vi "DangerEnemy.vi"(0 "MarkerSkill in":refnum<class "MarkerSkill.lvclass">, 5 "Game":refnum<class "Game.lvclass">, 11 "error in (no error)":errorcluster) -> (3 "Numero de inimigos\npossiveis para marcar":i32, 4 "MarkerSkill out":refnum<class "MarkerSkill.lvclass">, 6 "id do inimigo\nmais perigoso":u32, 8 "Pos do inimigo\nperigoso":dbl[](array[numeric]), 10 "id do segundo inimigo\nmais perigoso":i32, 13 "Id do Inimigo Mais Próximo":u32, 14 "Pos do segundo inimigo\nperigoso":dbl[](array[numeric]), 15 "error out":errorcluster)   [LabVIEW 2018, in "MarkerSkill.lvclass"]
uses:
  MarkerSkill.lvclass
  Game_class/Game.lvclass
  Game_class/Game.lvclass/Game.ctl
  Referee_class/Referee.lvclass/Referee.ctl
  Team_class/Team.lvclass/Team.ctl
  Object_class/Object.lvclass/Object.ctl
  Robot_class/Robot.lvclass/Robot.ctl
  Object_class/Read x.vi
  Object_class/Read y.vi
  Robot_class/Read id.vi
  <vilib>/Analysis/_algsub.llb/Real Vector Norm.vi
  Game_class/Read Referee.vi
  Game_class/Read EnemyRef.vi
  Game_class/Read FieldRef.vi
  Game_class/Read BallRef.vi
  Team_class/Read RobotRef.vi
  Referee_class/Read enemy_goalie_id.vi
  Enemy_class/Enemy.lvclass
  C:/Users/Gustavo/Desktop/RoboIME/SimplePass/SSL_AI/Team_class/Team.lvclass
  Ball_class/Ball.lvclass
  C:/Users/Gustavo/Desktop/RoboIME/SimplePass/SSL_AI/Object_class/Object.lvclass
  Robot_class/Robot.lvclass
  Referee_class/Referee.lvclass
  Field_class/Field.lvclass
  <vilib>/Analysis/NI_AALPro.lvlib
panel:
  in  "D para nao marcar":dbl=200.0
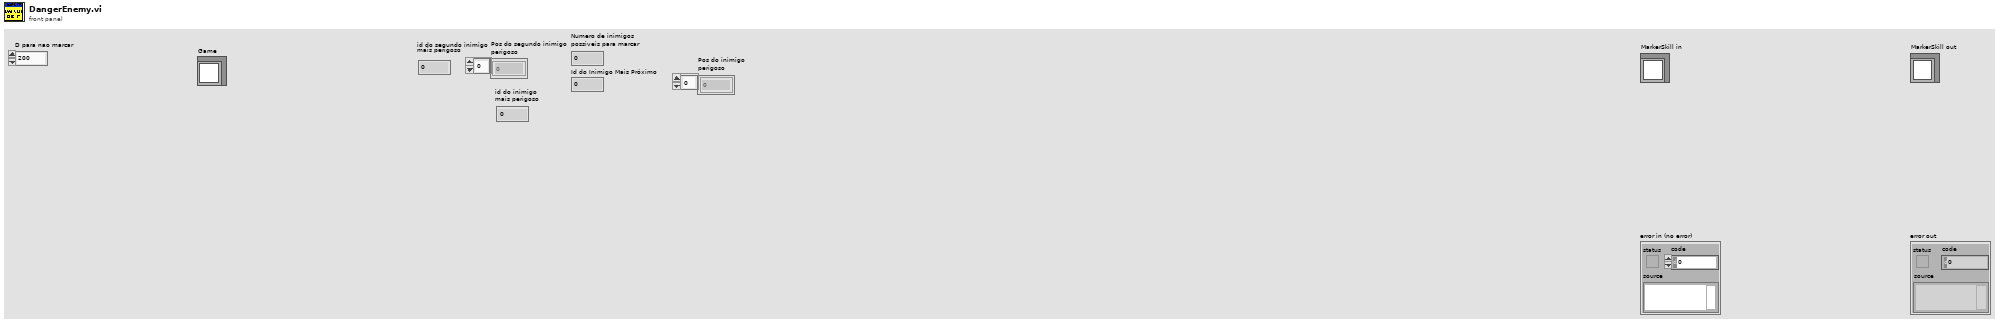
[diagram p1: front panel]
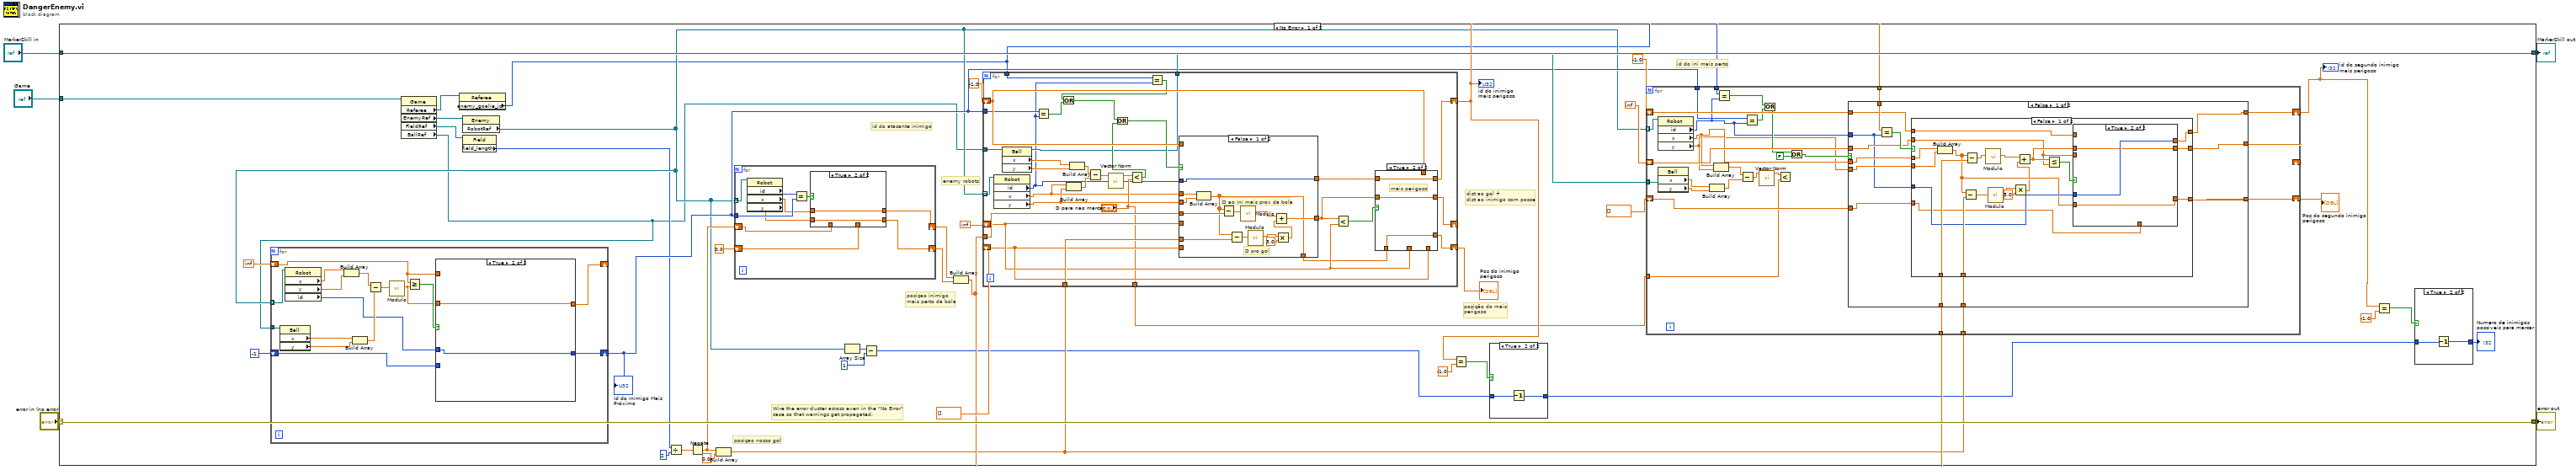
[diagram p0: block diagram]
diagram:
  n1 = case shown="No Error" "error in (no error)" {
    selector: "error in (no error)" -> [w47 w217]
    tunnel: [w47 w217] -> w4
    tunnel: [w48 w216] -> w2
    tunnel: "MarkerSkill in" -> [w48 w216]
    tunnel: "Game" -> [w6 _]
    frame No Error {
      # "id do ini mais perto"
      # "id do atacante inimigo"
      # "enemy robots"
      # "dist ao gol +\ndist ao inimigo com posse"
      # "posição do mais\nperigoso"
      # "posiçao nosso gol"
      # "posiçao inimigo\nmais perto da bola"
      # "Wire the error cluster across even in the \"No Error\"\ncase so that warnings get propagated."
      n2 = property class="Game"(reference=w6) -> ("Referee"=w8:refnum<class "Referee.lvclass">, "EnemyRef"=w13:refnum<class "Enemy.lvclass">, "FieldRef"=w12:refnum<class "Field.lvclass">, "BallRef"=w9:refnum<class "Ball.lvclass">)  [unwired: 1 in, 2 out]
      n3 = property class="Referee"(reference=w8) -> ("enemy_goalie_id"=w7:i32)  [unwired: 1 in, 2 out]
      n4 = property class="Enemy"(reference=w13) -> ("RobotRef"=w11:refnum<class "Robot.lvclass">[])  [unwired: 1 in, 2 out]
      n5 = for {
        tunnel: w11 -> [w58] mode=indexing
        tunnel: w9 -> [w61]
        shift-right: [w65] -> _
        shift-left: inf -> [w63]
        shift-right: [w64] -> w15
        shift-left: -1 -> [w62]
        n6 = property class="Ball"(reference=w61) -> ("x"=w60:dbl, "y"=w59:dbl)  [unwired: 1 in, 2 out]
        n7 = property class="Robot"(reference=w58) -> ("x"=w57:dbl, "y"=w56:dbl, "id"=w55:i32)  [unwired: 1 in, 2 out]
        n8 = Build Array(w57, w56) -> (w70:dbl[])
        n9 = Build Array(w60, w59) -> (w69:dbl[])
        n10 = Subtract(x=w70, y=w69) -> (x-y=w67:dbl[])
        n11 = call "Modulo.vi"("2D vector"=w67) -> ("Modulo"=w66:dbl)  [unwired: 10 in]
        n12 = Greater Or Equal?(x=w63, y=w66) -> (x >= y?=w68:bool)
        n13 = case shown="True" w68 {
          tunnel: [w72 w74] -> w65
          tunnel: w66 -> [_ w74]
          tunnel: w55 -> [_ w73]
          tunnel: [w71 w73] -> w64
          tunnel: w63 -> [w72 _]
          tunnel: w62 -> [w71 _]
          frame False {
          }
          frame True {
          }
        }
      }
      "Id do Inimigo Mais Próximo" <- w15
      n14 = property class="Field"(reference=w12) -> ("field_length"=w10:i32)  [unwired: 1 in, 2 out]
      n15 = Divide(x=w10, y=u32 2) -> (x/y=w44:dbl)
      n16 = Negate(x=w44) -> (-x=w39:dbl)
      n17 = Build Array(w39, 0.0 ("element")) -> (w33:dbl[])
      n18 = for {
        tunnel: w11 -> [w205] mode=indexing
        tunnel: w15 -> [w211]
        shift-right: [w209] -> w17
        shift-left: w39 -> [w207]
        shift-right: [w208] -> w46
        shift-left: 0.0 ("y") -> [w206]
        n19 = property class="Robot"(reference=w205) -> ("id"=w204:i32, "x"=w203:dbl, "y"=w202:dbl)  [unwired: 1 in, 2 out]
        n20 = Equal?(x=w204, y=w211) -> (x = y?=w210:bool)
        n21 = case shown="True" w210 {
          tunnel: w203 -> [_ w215]
          tunnel: w202 -> [_ w214]
          tunnel: [w213 w215] -> w209
          tunnel: [w212 w214] -> w208
          tunnel: w207 -> [w213 _]
          tunnel: w206 -> [w212 _]
          frame False {
          }
          frame True {
          }
        }
      }
      n22 = Array Size(array=w11) -> (size(s)=w30:i32)
      n23 = Subtract(x=w30, y=1) -> (x-y=w25:i32)
      n24 = Build Array(w17, w46) -> (w34:dbl[])
      n25 = for {
        tunnel: w11 -> [w151] mode=indexing
        tunnel: w34 -> [w179]
        tunnel: w33 -> [w178]
        shift-right: [w175] -> _
        shift-left: inf -> [w174]
        shift-right: [w172] -> w28
        shift-left: -1.0 ("id") -> [w169]
        shift-right: [w170] -> w42
        shift-left: dbl[] [] -> [w168]
        tunnel: w7 -> [w167]
        tunnel: w9 -> [w155]
        tunnel: [w152] -> w19
        tunnel: ["D para nao marcar"] -> w18
        tunnel: w15 -> [w157]
        n26 = property class="Robot"(reference=w151) -> ("id"=w148:i32, "x"=w150:dbl, "y"=w149:dbl)  [unwired: 1 in, 2 out]
        n27 = property class="Ball"(reference=w155) -> (reference out=w152:refnum<class "Ball.lvclass">, "x"=w154:dbl, "y"=w153:dbl)  [unwired: 1 in, 1 out]
        n28 = Equal?(x=w157, y=w148) -> (x = y?=w165:bool)
        n29 = Build Array(w150, w149) -> (w163:dbl[])
        n30 = Build Array(w154, w153) -> (w164:dbl[])
        n31 = Subtract(x=w164, y=w163) -> (x-y=w162:dbl[])
        n32 = call-poly <vilib>:"Vector Norm.vi"("Input Vector"=w162) -> ("norm"=w161:dbl)  [unwired: 9 in, 1 out]
        n33 = Less?(x=w161, y="D para nao marcar") -> (x < y?=w156:bool)
        n34 = Equal?(x=w167, y=w148) -> (x = y?=w166:bool)
        n35 = Or(x=w166, y=w165) -> (x .or. y?=w160:bool)
        n36 = Or(x=w160, y=w156) -> (x .or. y?=w159:bool)
        n37 = case shown="False" w159 {
          tunnel: w150 -> [w198 _]
          tunnel: w149 -> [w197 _]
          tunnel: w179 -> [w196 _]
          tunnel: w178 -> [w194 _]
          tunnel: [w191 w201] -> w176
          tunnel: w174 -> [_ w201]
          tunnel: w148 -> [w190 _]
          tunnel: [w190 w200] -> w173
          tunnel: [w189 w199] -> w171
          tunnel: w169 -> [_ w200]
          tunnel: w168 -> [_ w199]
          frame False {
            # "D ao ini mais prox da bola"
            # "D pro gol"
            n38 = Build Array(w198, w197) -> (w189:dbl[])
            n39 = Subtract(x=w189, y=w196) -> (x-y=w195:dbl[])
            n40 = Subtract(x=w189, y=w194) -> (x-y=w193:dbl[])
            n41 = call "Modulo.vi"("2D vector"=w195) -> ("Modulo"=w192:dbl)  [unwired: 10 in]
            n42 = call "Modulo.vi"("2D vector"=w193) -> ("Modulo"=w188:dbl)  [unwired: 10 in]
            n43 = Multiply(x=w188, y=3.0) -> (x*y=w186:dbl)
            n44 = Add(x=w192, y=w186) -> (x+y=w191:dbl)
          }
          frame True {
          }
        }
        n45 = Less?(x=w176, y=w174) -> (x < y?=w177:bool)
        n46 = case shown="True" w177 {
          tunnel: w176 -> [_ w185]
          tunnel: [w182 w185] -> w175
          tunnel: w174 -> [w182 _]
          tunnel: [w181 w184] -> w172
          tunnel: w173 -> [_ w184]
          tunnel: w169 -> [w181 _]
          tunnel: w171 -> [_ w183]
          tunnel: [w180 w183] -> w170
          tunnel: w168 -> [w180 _]
          frame False {
          }
          frame True {
            # "mais perigoso"
          }
        }
      }
      "id do inimigo\nmais perigoso" <- w28
      "Pos do inimigo\nperigoso" <- w42
      n47 = Equal?(x=w28, y=-1.0) -> (x = y?=w26:bool)
      n48 = case shown="True" w26 {
        tunnel: w25 -> [w52 w54]
        tunnel: [w52 w53] -> w21
        frame False {
        }
        frame True {
          n49 = Decrement(x=w54) -> (x-1=w53:i32)
        }
      }
      n50 = for {
        tunnel: w11 -> [w81] mode=indexing
        shift-right: [w102] -> w23
        shift-left: -1.0 -> [w101]
        shift-right: [w100] -> _
        shift-left: inf -> [w94]
        shift-right: [w99] -> w35
        shift-left: dbl[] [] -> [w98]
        tunnel: w28 -> [w97]
        tunnel: w34 -> [w96]
        tunnel: w33 -> [w95]
        tunnel: w7 -> [w93]
        tunnel: w19 -> [w77]
        tunnel: w18 -> [w86]
        tunnel: w15 -> [w83]
        n51 = property class="Robot"(reference=w81) -> ("id"=w80:i32, "x"=w79:dbl, "y"=w78:dbl)  [unwired: 1 in, 2 out]
        n52 = property class="Ball"(reference=w77) -> ("x"=w76:dbl, "y"=w75:dbl)  [unwired: 1 in, 2 out]
        n53 = Build Array(w76, w75) -> (w89:dbl[])
        n54 = Build Array(w79, w78) -> (w90:dbl[])
        n55 = Equal?(x=w93, y=w80) -> (x = y?=w92:bool)
        n56 = Subtract(x=w90, y=w89) -> (x-y=w88:dbl[])
        n57 = Equal?(x=w83, y=w80) -> (x = y?=w91:bool)
        n58 = call-poly <vilib>:"Vector Norm.vi"("Input Vector"=w88) -> ("norm"=w87:dbl)  [unwired: 9 in, 1 out]
        n59 = Or(x=w92, y=w91) -> (x .or. y?=w85:bool)
        n60 = Less?(x=w87, y=w86) -> ()  [unwired: 1 out]
        n61 = Or(x=w85, y=FALSE) -> (x .or. y?=w84:bool)
        n62 = case shown="False" w84 {
          tunnel: w101 -> [w113 w147]
          tunnel: [w112 w147] -> w102
          tunnel: w94 -> [w111 w146]
          tunnel: [w110 w146] -> w100
          tunnel: w98 -> [w109 w145]
          tunnel: [w108 w145] -> w99
          tunnel: w80 -> [w103 _]
          tunnel: w97 -> [w115 _]
          tunnel: w79 -> [w107 _]
          tunnel: w78 -> [w106 _]
          tunnel: w96 -> [w105 _]
          tunnel: w95 -> [w104 _]
          frame False {
            n63 = Equal?(x=w115, y=w103) -> (x = y?=w114:bool)
            n64 = case shown="False" w114 {
              tunnel: [w127 w144] -> w112
              tunnel: w113 -> [w125 w144]
              tunnel: w111 -> [w119 w143]
              tunnel: [w123 w143] -> w110
              tunnel: w109 -> [w120 w142]
              tunnel: [w121 w142] -> w108
              tunnel: w107 -> [w135 _]
              tunnel: w106 -> [w134 _]
              tunnel: w105 -> [w133 _]
              tunnel: w104 -> [w130 _]
              tunnel: w103 -> [w126 _]
              frame False {
                n65 = Build Array(w135, w134) -> (w122:dbl[])
                n66 = Subtract(x=w122, y=w130) -> (x-y=w129:dbl[])
                n67 = Subtract(x=w122, y=w133) -> (x-y=w132:dbl[])
                n68 = call "Modulo.vi"("2D vector"=w132) -> ("Modulo"=w131:dbl)  [unwired: 10 in]
                n69 = call "Modulo.vi"("2D vector"=w129) -> ("Modulo"=w118:dbl)  [unwired: 10 in]
                n70 = Multiply(x=w118, y=3.0) -> (x*y=w116:dbl)
                n71 = Add(x=w131, y=w116) -> (x+y=w124:dbl)
                n72 = Less Or Equal?(x=w124, y=w119) -> (x <= y?=w128:bool)
                n73 = case shown="True" w128 {
                  tunnel: [w138 w141] -> w127
                  tunnel: w126 -> [_ w141]
                  tunnel: w125 -> [w138 _]
                  tunnel: [w136 w140] -> w123
                  tunnel: w124 -> [_ w140]
                  tunnel: [w137 w139] -> w121
                  tunnel: w122 -> [_ w139]
                  tunnel: w120 -> [w137 _]
                  tunnel: w119 -> [w136 _]
                  frame False {
                  }
                  frame True {
                  }
                }
              }
              frame True {
              }
            }
          }
          frame True {
          }
        }
      }
      "id do segundo inimigo\nmais perigoso" <- w23
      "Pos do segundo inimigo\nperigoso" <- w35
      n74 = Equal?(x=w23, y=-1.0) -> (x = y?=w22:bool)
      n75 = case shown="True" w22 {
        tunnel: w21 -> [w49 w51]
        tunnel: [w49 w50] -> w20
        frame False {
        }
        frame True {
          n76 = Decrement(x=w51) -> (x-1=w50:i32)
        }
      }
      "Numero de inimigos\npossiveis para marcar" <- w20
    }
    frame Error {
    }
  }
  "error out" <- w4
  "MarkerSkill out" <- w2
